vi "gardner.vi"(0 "in":cdb[](array[numeric]), 11 "sps":dbl=8.0) -> (4 "sym":cdb[](array[numeric]), 15 "offsetvec":dbl[](array[numeric]))   [LabVIEW 2013]
uses:
  <vilib>/imath/engines/lvmath2/RunTimeEngine/ErrorHandling/NIMS_Finalize Error.vi
  <vilib>/imath/engines/lvmath2/RunTimeEngine/Managers/WorkSpace/UID Generator.vi
  <vilib>/imath/engines/lvmath2/RunTimeEngine/Managers/SymbolTable/Clear UID.vi
  <vilib>/imath/engines/lvmath2/RunTimeEngine/NodeEndStatement/NIMS_NodeEndStatement_Output.vi
  <instcachedir>/0/NIMS_NodeEndStatement_Output_53EC0D466D134D7ABD903AC30B43404B.lvgen/NIMS_NodeEndStatement_Output_53EC0D466D134D7ABD903AC30B43404B_005.vi
  <instcachedir>/0/NIMS_NodeEndStatement_Output_53EC0D466D134D7ABD903AC30B43404B.lvgen/NIMS_NodeEndStatement_Output_53EC0D466D134D7ABD903AC30B43404B_000.vi
  LabVIEW Data/MathScriptVIs/MCStatic_31879994332_7f37ed9731ed4f5c5ae0d9a3646a6e9e.vi
  <instcachedir>/0/MCStatic_31879994332_7f37ed9731ed4f5c5ae0d9a3646a6e9e_2FF9FAA442424E60824EA660B4DC2294.lvgen/MCStatic_31879994332_7f37ed9731ed4f5c5ae0d9a3646a6e9e_2FF9FAA442424E60824EA660B4DC2294_000.vi
  MATLAB_func/gardner_symbol_recovery.m
  <vilib>/imath/engines/lvmath2/RunTimeEngine/Managers/SymbolTable/NIMS_WorkSpace.lvlib
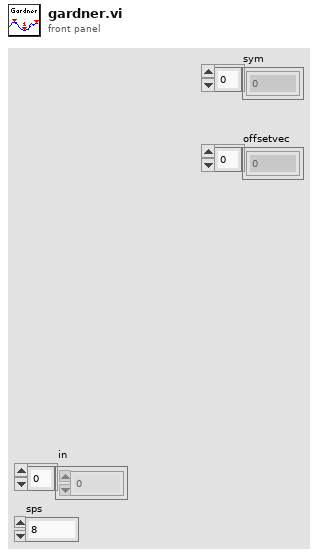
[diagram p1: front panel]
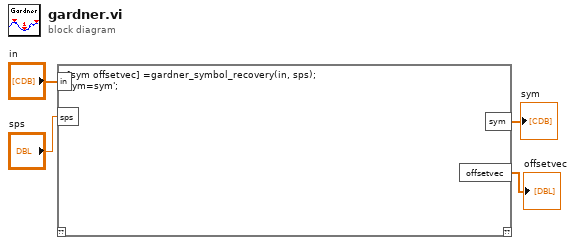
[diagram p0: block diagram]
diagram:
  n1 = mathscript code="[sym offsetvec] =gardner_symbol_recovery(in, sps);\nsym=sym';"("in"="in", "sps"="sps") -> ("sym"=→"sym":cdb[], "offsetvec"=→"offsetvec":dbl[])  [unwired: 1 in, 1 out]
